vi "Get Connection List.vi"(8 "error in (no error)":errorcluster, 11 "PIPXI40 Matrix in":refnum<class "PIPX40 Matrix.lvclass">) -> (0 "error out":errorcluster, 2 "List":variant, 3 "PIPXI40 Matrix out":refnum<class "PIPX40 Matrix.lvclass">)   [LabVIEW 2020, in "Pickering.lvlib" / "PIPX40 Matrix.lvclass"]
uses:
  PIPX40 Matrix.lvclass
  D:/WSGitHub/RTFWK/Realization/PIPX40 Base/PIPX40 Base.lvclass
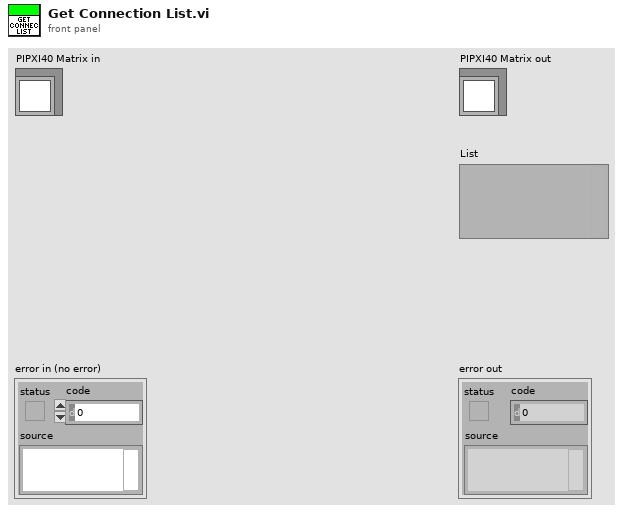
[diagram p1: front panel]
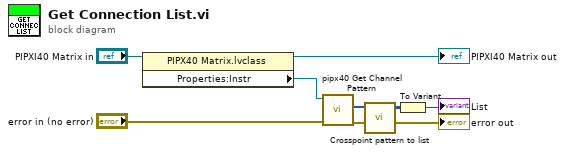
[diagram p0: block diagram]
diagram:
  n1 = property class="PIPX40 Matrix.lvclass"(reference="PIPXI40 Matrix in") -> (reference out=→"PIPXI40 Matrix out":refnum<class "PIPX40 Matrix.lvclass">, "Properties:Instr"=w5:refnum<visa-resource-name>)  [unwired: 1 in, 1 out]
  n2 = call <instrlib>:"pipx40 Get Channel Pattern.vi"("error in (no error)"="error in (no error)", "instrument handle"=w5) -> ("error out"=→"error out":errorcluster, "pattern"=w3:u32[])  [unwired: 7 in, 1 out]
  n3 = call "Crosspoint pattern to list.vi"("Pattern"=w3) -> ("List"=w1:i32[][])  [unwired: 10 in]
  n4 = To Variant(anything=w1) -> (Variant=→"List":variant)
